vi "SRS 830 Ramp Freq.vi"(2 "Point #":i32, 4 "Parameters":dbl[](array[numeric]) format="%.3e", 5 "Instrument Address":refnum<visa-resource-name>) -> (0 "Stop":bool, 1 "Data Out":dbl[](array[numeric]) format="%.2e")   [LabVIEW 2019]
doc: "This VI reads the sample output of the Lakeshore DRC 93C or 82C temperature controller. The output is an array consisting of the single reading. The input is the numeric GPIB address.\nScott Hannahs, F. Bitter National Magnet Lab, 1993"
panel:
  # "Starting Freq"
  # "Ending Freq"
  # "Time (Min)"
  # "Log (>0)"
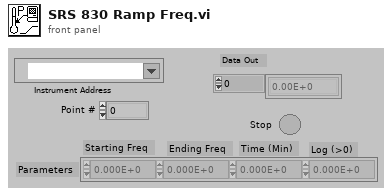
[diagram p1: front panel]
types:
  T1 = cluster{"Parameters[0]":dbl, "Parameters[1]":dbl, "Parameters[2]":dbl, "Parameters[3]":dbl}
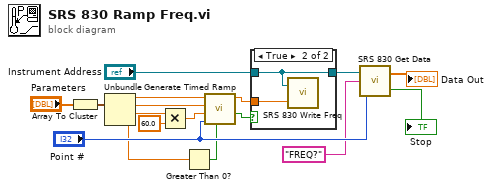
[diagram p0: block diagram]
diagram:
  n1 = Array To Cluster(array="Parameters") -> (cluster=w16:T1)
  n2 = Unbundle(w16) -> ("Parameters[0]"=w11:dbl, "Parameters[1]"=w10:dbl, "Parameters[2]"=w9:dbl, "Parameters[3]"=w3:dbl)
  n3 = Multiply(x=w9, y=60.0) -> (x*y=w2:dbl)
  n4 = Greater Than 0?(x=w3) -> (x > 0?=w4:bool)
  n5 = call "Generate Timed Ramp.vi"("Log"=w4, "Point #"="Point #", "Time (Hr:Min:Sec)"=w2, "Stop"=w10, "Start"=w11) -> ("Valid"=w7:bool, "Output"=w8:dbl)  [unwired: 2 out]
  n6 = case shown="True" w7 {
    tunnel: "Instrument Address" -> [w18 w19]
    tunnel: w8 -> [_ w20]
    tunnel: [w18 w19] -> w5
    frame False {
    }
    frame True {
      n7 = call "SRS 830 Write Freq.vi"("Setpoint"=w20, "Instrument Address"=w19) -> ()  [unwired: 1 in]
    }
  }
  n8 = call "SRS 830 Get Data.vi"("Point #"="Point #", "Command String"="FREQ?", "Instrument Address"=w5) -> ("Stop"=→"Stop":bool, "SRS 830 Output"=→"Data Out":dbl[])
